vi "Open App Reference.vi"(8 "error in (no error)":errorcluster, 11 "App Instance":T1) -> (0 "error out":errorcluster, 2 "VI Server Configured?":bool, 3 "App Ref":refnum<vi>)   [LabVIEW 2020, in "MacroAssert.lvlib"]
doc: "Opens and outputs an application reference to the application instance defined by <B>App Instance</B>."
uses:
  MacroAssert.lvlib
  CTLs/App Instance.ctl
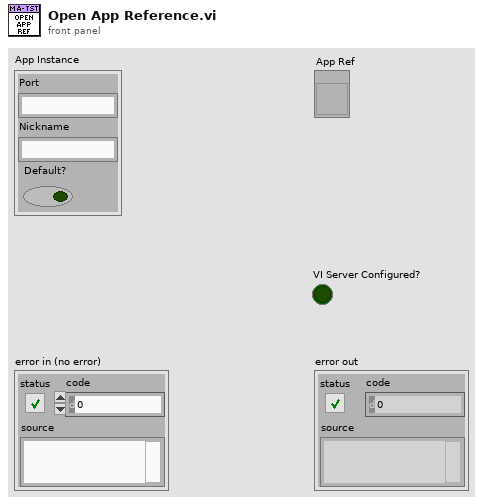
[diagram p1: front panel]
types:
  T1 = typedef "MacroAssert.lvlib/App Instance.ctl" = cluster{"Port":string, "Nickname":string, "Default?":bool}
  T2 = enum32{"invalid app kind", "Development System", "Run Time System", "Student Edition", "Embedded LabVIEW", "Evaluation", "Custom"}
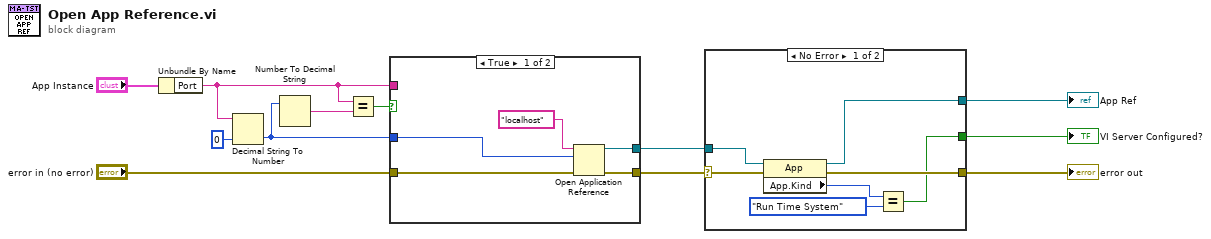
[diagram p0: block diagram]
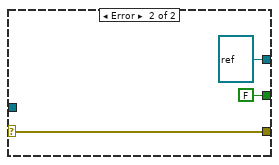
[diagram p2: hidden frame]
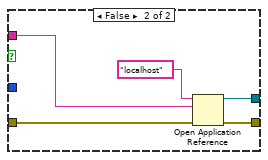
[diagram p3: hidden frame]
diagram:
  n1 = Unbundle By Name("App Instance") -> ("Port"=w7:string)
  n2 = Decimal String To Number(string=w7, default (0L)=u16 0 ("default (0 I32)")) -> (number=w9:u16)  [unwired: 1 in, 1 out]
  n3 = Number To Decimal String(number=w9) -> (decimal integer string=w10:string)  [unwired: 1 in]
  n4 = Equal?(x=w7, y=w10) -> (x = y?=w8:bool)
  n5 = case shown="True" w8 {
    tunnel: "error in (no error)" -> [w17 w22]
    tunnel: [w15 w20] -> w5
    tunnel: [w14 w19] -> w4
    tunnel: w9 -> [w13 _]
    tunnel: w7 -> [_ w18]
    frame True {
      n6 = Open Application Reference(8:w17, 10:w13, 11:"localhost" ("machine name (\"\":  open local reference)")) -> (0:w15:errorcluster, 3:w14:refnum<vi>)  [unwired: 1 in]
    }
    frame False {
      n7 = Open Application Reference(8:w22, 10:w18, 11:"localhost" ("machine name (\"\":  open local reference)")) -> (0:w20:errorcluster, 3:w19:refnum<vi>)  [unwired: 1 in]
    }
  }
  n8 = case shown="No Error" w5 {
    selector: w5 -> [w29 w32]
    tunnel: w4 -> [w28 _]
    tunnel: [w27 w32] -> w3
    tunnel: [w26 refnum<vi> refnum ("application reference")] -> w2
    tunnel: [w23 FALSE] -> w1
    frame No Error {
      n9 = property class="App"(reference=w28, error in=w29) -> (reference out=w26:refnum<vi>, error out=w27:errorcluster, "App.Kind"=w25:T2)
      n10 = Equal?(x=w25, y=T2."Run Time System") -> (x = y?=w23:bool)
    }
    frame Error {
    }
  }
  "error out" <- w3
  "App Ref" <- w2
  "VI Server Configured?" <- w1
